vi "stitch interpolated images.vi"(9 "DeltaE":dbl, 10 "Array of images to stitch":cluster{dbl[][]}[](array[cluster]), 11 "calib \"final\"":T1[](array[typedef])) -> (3 "stitched array image":sgl[][](array[numeric]))   [LabVIEW 2020, in "MagSpec_Bella.lvclass"]
uses:
  MagSpec_Bella.lvclass
  finalCalib--Cluster.ctl
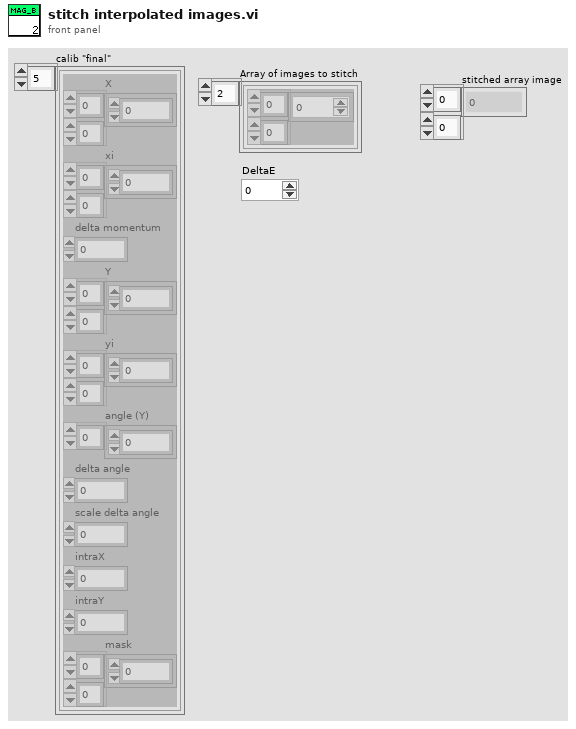
[diagram p1: front panel]
types:
  T1 = typedef "finalCalib--Cluster.ctl" = cluster{"X":dbl[][], "xi":dbl[][], "delta momentum":dbl, "Y":dbl[][], "yi":dbl[][], "angle (Y)":dbl[], "delta angle":dbl, "scale delta angle":dbl, "intraX":dbl, "intraY":dbl, "mask":dbl[][]}
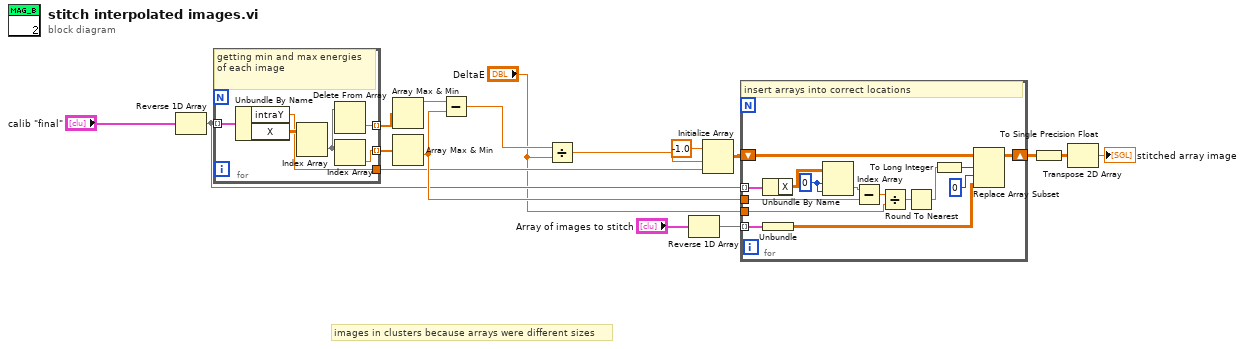
[diagram p0: block diagram]
diagram:
  # "images in clusters because arrays were different sizes"
  n1 = Reverse 1D Array(array="calib \"final\"") -> (reversed array=w10:T1[])
  n2 = for {
    tunnel: w10 -> [w23] mode=indexing
    tunnel: [w20] -> w5 mode=indexing
    tunnel: [w19] -> w4 mode=indexing
    tunnel: [w18] -> w8
    # "getting min and max energies of each image"
    n3 = Unbundle By Name(w23) -> ("intraY"=w18:dbl, "X"=w22:dbl[][])
    n4 = Index Array(array=w22) -> (element=w21:dbl[])  [unwired: 2 in]
    n5 = Delete From Array(array=w21) -> (deleted portion=w20:dbl)  [unwired: 2 in, 1 out]
    n6 = Index Array(array=w21) -> (element=w19:dbl)  [unwired: 1 in]
  }
  n7 = Array Max & Min(array=w5) -> (max value=w6:dbl)  [unwired: 3 out]
  n8 = Array Max & Min(array=w4) -> (min value=w12:dbl)  [unwired: 3 out]
  n9 = Subtract(x=w6, y=w12) -> (x-y=w16:dbl)
  n10 = Divide(x=w16, y="DeltaE") -> (x/y=w17:dbl)
  n11 = Reverse 1D Array(array="Array of images to stitch") -> (reversed array=w11:cluster{dbl[][]}[])
  n12 = Initialize Array(-1.0, w17, w8) -> (w9:dbl[][])
  n13 = for {
    tunnel: w10 -> [w35] mode=indexing
    tunnel: "DeltaE" -> [w29]
    shift-right: [w28] -> w13
    shift-left: w9 -> [w38]
    tunnel: w11 -> [w37] mode=indexing
    tunnel: w12 -> [w31]
    w33 = 0 ("disabled index (row)")
    # "insert arrays into correct locations"
    n14 = Unbundle By Name(w35) -> ("X"=w34:dbl[][])
    n15 = Unbundle(w37) -> (w36:dbl[][])
    n16 = Index Array(array=w34, index (row)=w33, index (col)=w33) -> (element=w32:dbl)
    n17 = Subtract(x=w32, y=w31) -> (x-y=w30:dbl)
    n18 = Divide(x=w30, y=w29) -> (x/y=w26:dbl)
    n19 = Round To Nearest(number=w26) -> (nearest integer value=w27:dbl)
    n20 = To Long Integer(number=w27) -> (32bit integer=w25:i32)
    n21 = Replace Array Subset(array=w38, new element=w36, index (row)=w25, index (col)=0 ("disabled index (row)")) -> (w28:dbl[][])
  }
  n22 = To Single Precision Float(number=w13) -> (single precision float=w14:sgl[][])
  n23 = Transpose 2D Array(2D array=w14) -> (transposed array=→"stitched array image":sgl[][])
